vi "O2 Leak FGV.vi"(6 "Aktion":T4, 7 "Protokoll":T1 {"Messgasdruck" format="%.1f"; "O2" format="%.1f"}, 8 "error in (no error)":errorcluster caption="Fehler (Eingang, kein Fehler)", 9 "Textname:":string, 10 "Pfad:":path=path "D:/IAG_Data/Log", 11 "O2 Settings":T2 {"Grenzwert: Messgasdruck 2" format="%#.1f"; "Grenzwert: Messgasdruck" format="%#.1f"; "Grenzwert: O2" format="%#.3f"; "Datenerfassungszeit:" format="%#.1f"; "Nullgas Aufschaltzeit:" format="%#.1f"; "Aufschaltpunkt" items=["Filterblock", "Analyzer directly", "PNS"]; "Kalibriergas" items=["Stickstoff", "CO", "C3H8", "CH4", "O2", "", "", "", "", "", "", "", ""]}) -> (0 "error out":errorcluster caption="Fehler (Ausgang)", 1 "Textname:":string, 2 "Pfad:":path, 3 "O2 Settings":T2 {"Grenzwert: Messgasdruck 2" format="%#.1f"; "Grenzwert: Messgasdruck" format="%#.1f"; "Grenzwert: O2" format="%#.3f"; "Datenerfassungszeit:" format="%#.1f"; "Nullgas Aufschaltzeit:" format="%#.1f"; "Aufschaltpunkt" items=["Filterblock", "Analyzer directly", "PNS"]; "Kalibriergas" items=["Stickstoff", "CO", "C3H8", "CH4", "O2", "", "", "", "", "", "", "", ""]}, 5 "Protokoll":T1 {"Messgasdruck" format="%.1f"; "O2" format="%.1f"})   [LabVIEW 2020, in "O2 Dichtheitstest.lvlib"]
uses:
  O2 Dichtheitstest.lvlib
  Aktion FGV O2 Leak.ctl
  O2 Settings.ctl
  Visualisierungs Elemente/Auswahlfeld.ctl
  Protokoll LeakTest.ctl
  Allgemein/allgemeine Sub-VIs.lvlib
panel:
  # "-"
  # "-"
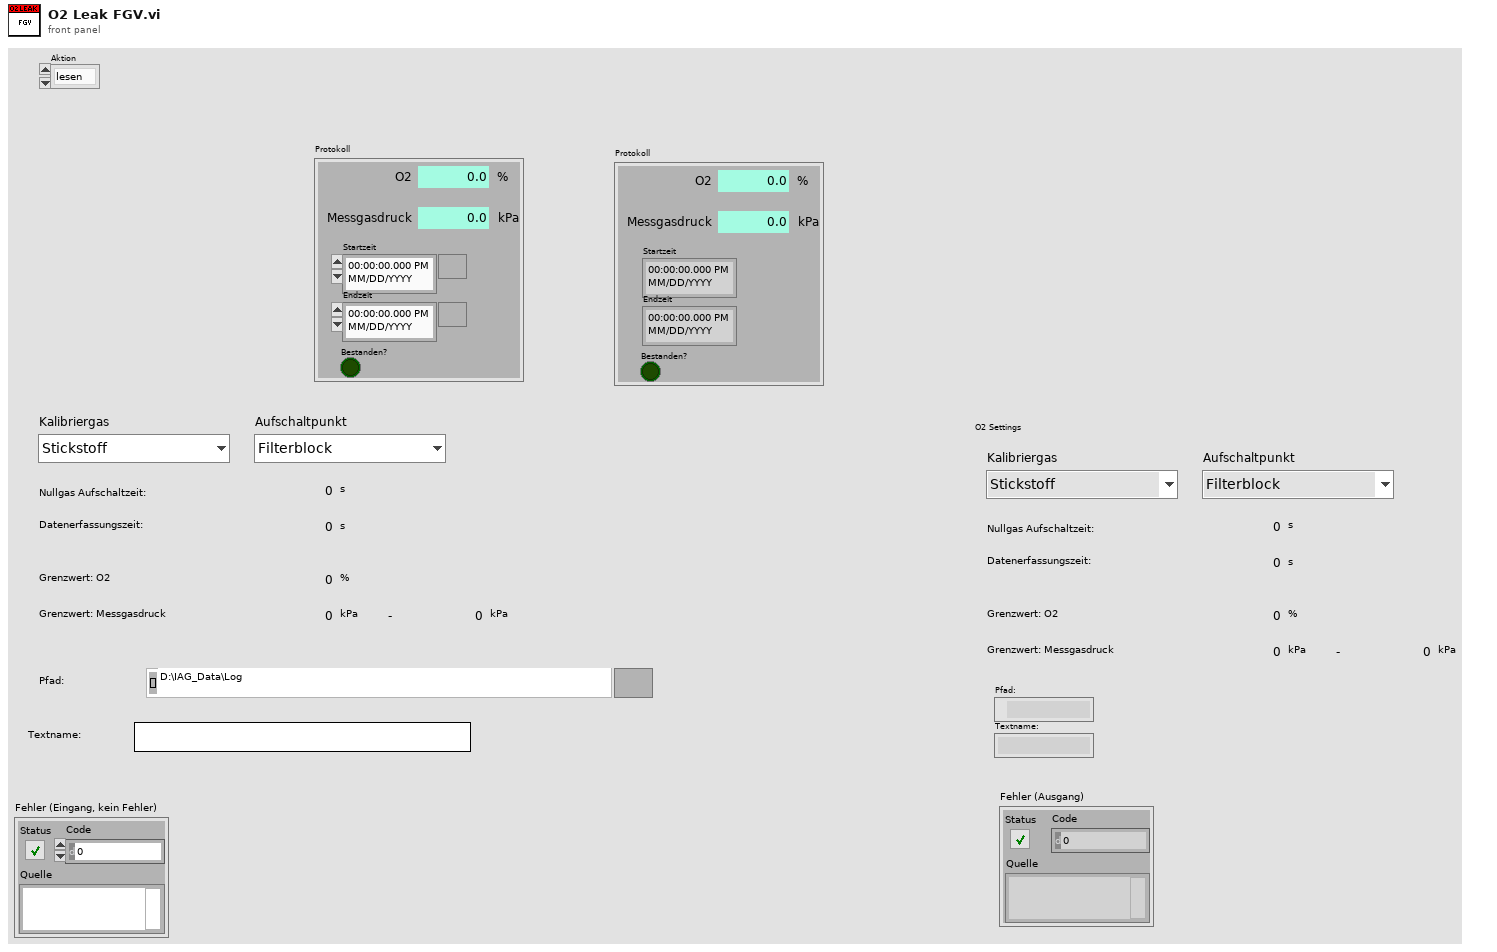
[diagram p1: front panel]
types:
  T1 = typedef "O2 Dichtheitstest.lvlib/Protokoll LeakTest.ctl" = cluster{"O2":sgl, "Messgasdruck":sgl, "Startzeit":timestamp, "Endzeit":timestamp, "Bestanden?":bool}
  T2 = typedef "O2 Dichtheitstest.lvlib/O2 Settings.ctl" = cluster{"Kalibriergas":T3, "Aufschaltpunkt":T3, "Nullgas Aufschaltzeit:":sgl, "Datenerfassungszeit:":sgl, "Grenzwert: O2":sgl, "Grenzwert: Messgasdruck":sgl, "Grenzwert: Messgasdruck 2":sgl}
  T3 = typedef "Auswahlfeld.ctl" = u16
  T4 = typedef "O2 Dichtheitstest.lvlib/Aktion FGV O2 Leak.ctl" = enum16{"lesen", "O2 settings", "Pfad", "Protokoll", "laden", "speichern"}
  T5 = cluster{"O2 Settings":T2, "Textname:":string, "Pfad:":path}
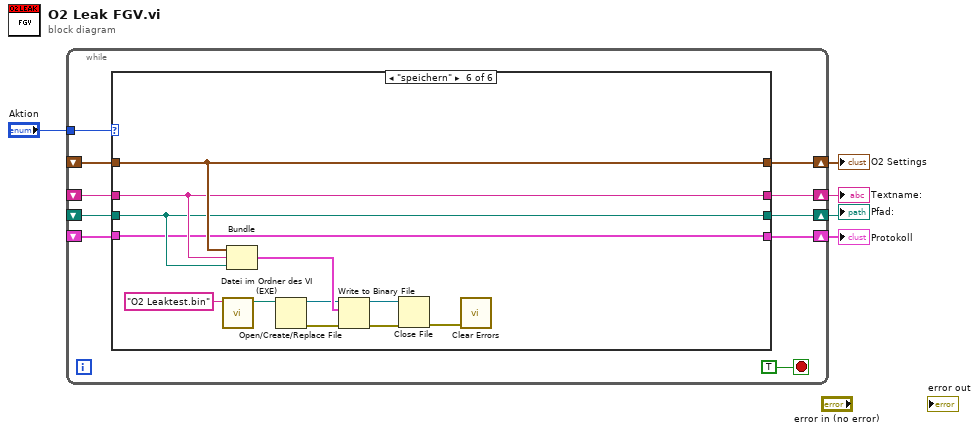
[diagram p0: block diagram]
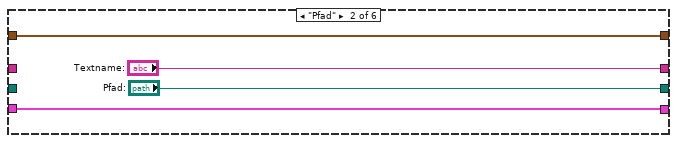
[diagram p3: hidden frame]
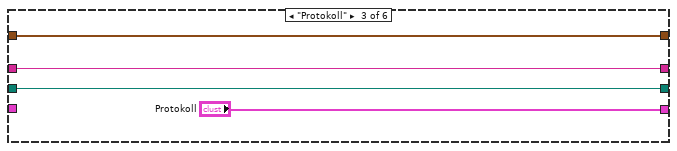
[diagram p4: hidden frame]
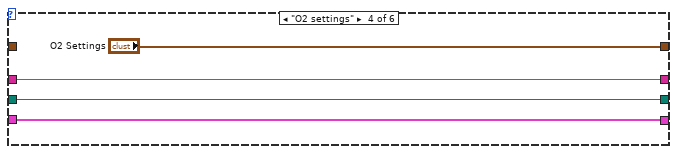
[diagram p5: hidden frame]
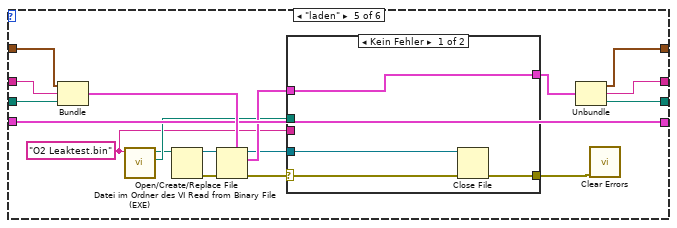
[diagram p6: hidden frame]
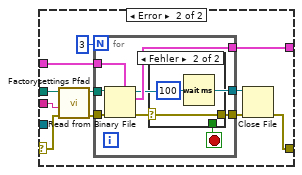
[diagram p7: hidden frame]
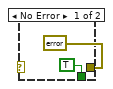
[diagram p8: hidden frame]
diagram:
  n1 = while {
    tunnel: "Aktion" -> [w15]
    shift-right: [w14] -> w4
    shift-left: _ -> [w13]
    shift-right: [w11] -> w2
    shift-left: _ -> [w9]
    shift-right: [w12] -> w3
    shift-left: _ -> [w10]
    shift-right: [w7] -> w1
    shift-left: _ -> [w6]
    stop <- TRUE stop-if-true
    n2 = case shown="\"speichern\"" w15 {
      tunnel: [w19 w23 w27 "O2 Settings" w45 w86] -> w14
      tunnel: w13 -> [w19 w23 w27 _ w48 w86]
      tunnel: [w18 "Textname:" w26 w30 w44 w85] -> w12
      tunnel: [w17 "Pfad:" w25 w29 w43 w84] -> w11
      tunnel: w10 -> [w18 _ w26 w30 w47 w85]
      tunnel: w9 -> [w17 _ w25 w29 w46 w84]
      tunnel: [w16 w20 "Protokoll" w28 w42 w83] -> w7
      tunnel: w6 -> [w16 w20 _ w28 w42 w83]
      frame "lesen", Default {
      }
      frame "Pfad" {
      }
      frame "Protokoll" {
      }
      frame "O2 settings" {
      }
      frame "laden" {
        w39 = "O2 Leaktest.bin" ("Dateiname")
        n3 = Bundle("O2 Settings"=w48, "Textname:"=w47, "Pfad:"=w46) -> (w49:T5)  [unwired: 1 in]
        n4 = call "Datei im Ordner des VI (EXE).vi"("Dateiname"=w39) -> ("Ordner des Haupt-VIs"=w40:path, "Dateipfad im Ordner des Haupt-VIs"=w33:path)  [unwired: 8 in, 1 out]
        n5 = Open/Create/Replace File(file path (use dialog)=w33) -> (refnum out=w32:refnum<file>, error out=w34:errorcluster)  [unwired: 5 in, 1 out]
        n6 = Read from Binary File(5:w49, 8:w34, 11:w32) -> (0:w37:errorcluster, 2:w41:T5, 3:w38:refnum<file>)  [unwired: 3 in, 1 out]
        n7 = case shown="Kein Fehler" w37 {
          selector: w37 -> [w52 w56]
          tunnel: w40 -> [_ w57]
          tunnel: w41 -> [w53 w55]
          tunnel: [w53 w63] -> w36
          tunnel: [w50 w61] -> w35
          tunnel: w38 -> [w51 _]
          tunnel: w39 -> [_ w54]
          frame No Error {
            n8 = Close File(refnum=w51, error in=w52) -> (error out=w50:errorcluster)  [unwired: 1 out]
          }
          frame Error {
            n9 = call "Factorysettings Pfad.vi"("error in (no error)"=w56, "Dateiname"=w54, "Ordner des Haupt-VIs"=w57) -> ("error out"=w58:errorcluster, "Pfad Factorysettings"=w59:path)  [unwired: 7 in]
            n10 = for {
              N: 3 -> [_]
              tunnel: w58 -> [w70]
              tunnel: w59 -> [w69]
              tunnel: [w68] -> w63
              tunnel: [w67] -> w62
              tunnel: [w66] -> w60
              tunnel: w55 -> [w65]
              stop <- w71 stop-if-true
              n11 = Read from Binary File(5:w65, 8:w70, 11:w69) -> (0:w72:errorcluster, 2:w68:T5, 3:w66:refnum<file>)  [unwired: 3 in, 1 out]
              n12 = case shown="Fehler" w72 {
                selector: w72 -> [_ w75]
                tunnel: [TRUE _] -> w71
                tunnel: [errorcluster {"status"=FALSE, "code"=0, "source"=""} ("error IO") w75] -> w67
                frame No Error {
                }
                frame Error {
                  n13 = Wait (ms)(milliseconds to wait=u32 100 ("Zu wartende ms")) -> ()  [unwired: 1 out]
                }
              }
            }
            n14 = Close File(refnum=w60, error in=w62) -> (error out=w61:errorcluster)  [unwired: 1 out]
          }
        }
        n15 = Unbundle(w36) -> ("O2 Settings"=w45:T2, "Textname:"=w44:string, "Pfad:"=w43:path)
        n16 = call <vilib>:"Clear Errors.vi"("error in (no error)"=w35) -> ()  [unwired: 5 in, 2 out]
      }
      frame "speichern" {
        n17 = call "Datei im Ordner des VI (EXE).vi"("Dateiname"="O2 Leaktest.bin") -> ("Dateipfad im Ordner des Haupt-VIs"=w82:path)  [unwired: 8 in, 2 out]
        n18 = Bundle("O2 Settings"=w86, "Textname:"=w85, "Pfad:"=w84) -> (w88:T5)  [unwired: 1 in]
        n19 = Open/Create/Replace File(file path (use dialog)=w82) -> (refnum out=w81:refnum<file>, error out=w80:errorcluster)  [unwired: 5 in, 1 out]
        n20 = Write to Binary File(file (use dialog)=w81, data=w88, error in=w80) -> (refnum out=w78:refnum<file>, error out=w79:errorcluster)  [unwired: 3 in, 1 out]
        n21 = Close File(refnum=w78, error in=w79) -> (error out=w77:errorcluster)  [unwired: 1 out]
        n22 = call <vilib>:"Clear Errors.vi"("error in (no error)"=w77) -> ()  [unwired: 5 in, 2 out]
      }
    }
  }
  "O2 Settings" <- w4
  "Textname:" <- w3
  "Pfad:" <- w2
  "Protokoll" <- w1
